vi "Read Operational Force Test Settings.vi"(8 "error in (no error)":errorcluster, 11 "Boot Loader in":refnum<class "Boot Loader.lvclass">) -> (0 "error out":errorcluster, 2 "Operational Force Test Settings":T1 {"Sample Time (s)" format="%.4f"; "Process Time (s)" format="%.4f"; "Max Force Error (N)" format="%.4f"}, 3 "Boot Loader out":refnum<class "Boot Loader.lvclass">)   [LabVIEW 2016, in "Boot Loader.lvclass"]
uses:
  Boot Loader.lvclass
  Typedefs/OperationalForceTestSettings.ctl
  Settings/Settings.lvclass
  Typedefs/FAMT Typedefs.lvlib
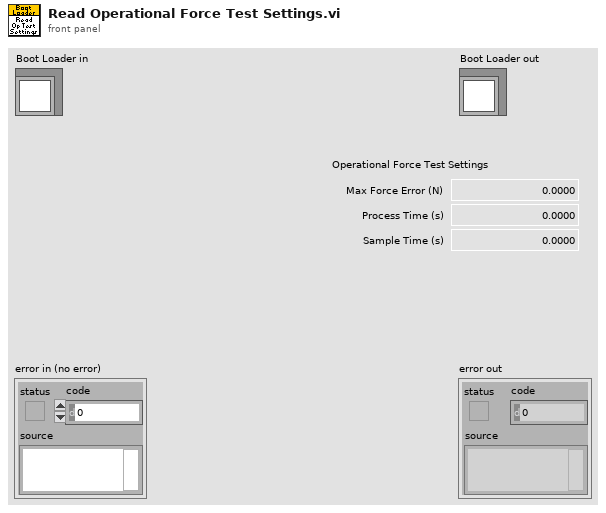
[diagram p1: front panel]
types:
  T1 = typedef "FAMT Typedefs.lvlib/OperationalForceTestSettings.ctl" = cluster{"Max Force Error (N)":dbl, "Process Time (s)":dbl, "Sample Time (s)":dbl}
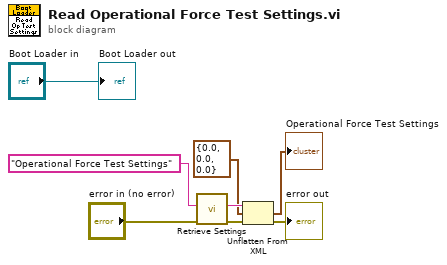
[diagram p0: block diagram]
diagram:
  n1 = call "Retrieve Settings.vi"("error in (no error)"="error in (no error)", "configName"="Operational Force Test Settings") -> ("error out"=w4:errorcluster, "xmlConfig"=w7:string)  [unwired: 7 in, 1 out]
  n2 = Unflatten From XML(xml string=w7, type=T1 {"Max Force Error (N)"=0.0, "Process Time (s)"=0.0, "Sample Time (s)"=0.0} ("Operational Force Test Settings"), error in (no error)=w4) -> (value=→"Operational Force Test Settings":T1, error out=→"error out":errorcluster)
  "Boot Loader out" <- "Boot Loader in"
